vi "Launcher.vi"   [LabVIEW 2019]
uses:
  #typedef_LauncherStates_enum.ctl
  #typedef_Queue_enum.ctl
  #typedef_Data_Entry.ctl
  #typedef_EntryConsole_Action_enum.ctl
  #typedef_Data_Cluster.ctl
  #typedef_WashDisplay_Action_enum.ctl
  #typedef_Controller_Action_enum.ctl
  #typedef_VehiclePosition_Action_enum.ctl
  #typedef_Data_Controller.ctl
types:
  T1 = typedef "#typedef_LauncherStates_enum.ctl" = enum16{"ERROR_default", "DefineCustomError", "InitIntermoduleQueues", "InitModules", "Run", "CloseIntermoduleQueues", "CloseApp"}
  T2 = typedef "#typedef_Queue_enum.ctl" = enum16{"ERROR_default", "Obtain", "Enqueue", "GetStatus", "Flush", "Release"}
  T3 = typedef "#typedef_Data_Controller.ctl" = cluster{"EntryConsole_Action":T4, "WashDisplay_Action":T5, "Controller_Action":T6, "VehiclePosition_Action":T7}
  T4 = typedef "#typedef_EntryConsole_Action_enum.ctl" = enum16{"Init", "ERROR_DEFAULT", "Idle", "Pending_Wash_Cycle", "Clear_Console", "Close", "Error_Handler", "Exit"}
  T5 = typedef "#typedef_WashDisplay_Action_enum.ctl" = enum16{"Init", "ERROR_DEFAULT", "Idle", "Specific", "Close", "Error_Handler", "Exit"}
  T6 = typedef "#typedef_Controller_Action_enum.ctl" = enum16{"Init", "ERROR_DEFAULT", "Idle", "Read database", "Close", "Error_Handler", "Exit"}
  T7 = typedef "#typedef_VehiclePosition_Action_enum.ctl" = enum16{"Init", "ERROR_DEFAULT", "Idle", "Specific", "Close", "Error_Handler", "Exit"}
  T8 = typedef "#typedef_Data_Cluster.ctl" = cluster{"Dummy":dbl, "EntryConsole_Action":T4, "WashDisplay_Action":T5, "Controller_Action":T6, "VehiclePosition_Action":T7}
  T9 = typedef "#typedef_Data_Entry.ctl" = cluster{"Under Body Wash":bool, "Bug Remover":bool, "Pre-Soak":bool, "High Pressure Wash (default)":bool, "Low Pressure Wax":bool, "Spot Free Rinse":bool, "Tire Shine Foam":bool, "Air Dry":bool, "Start":bool, "EntryConsole_Action":T4}
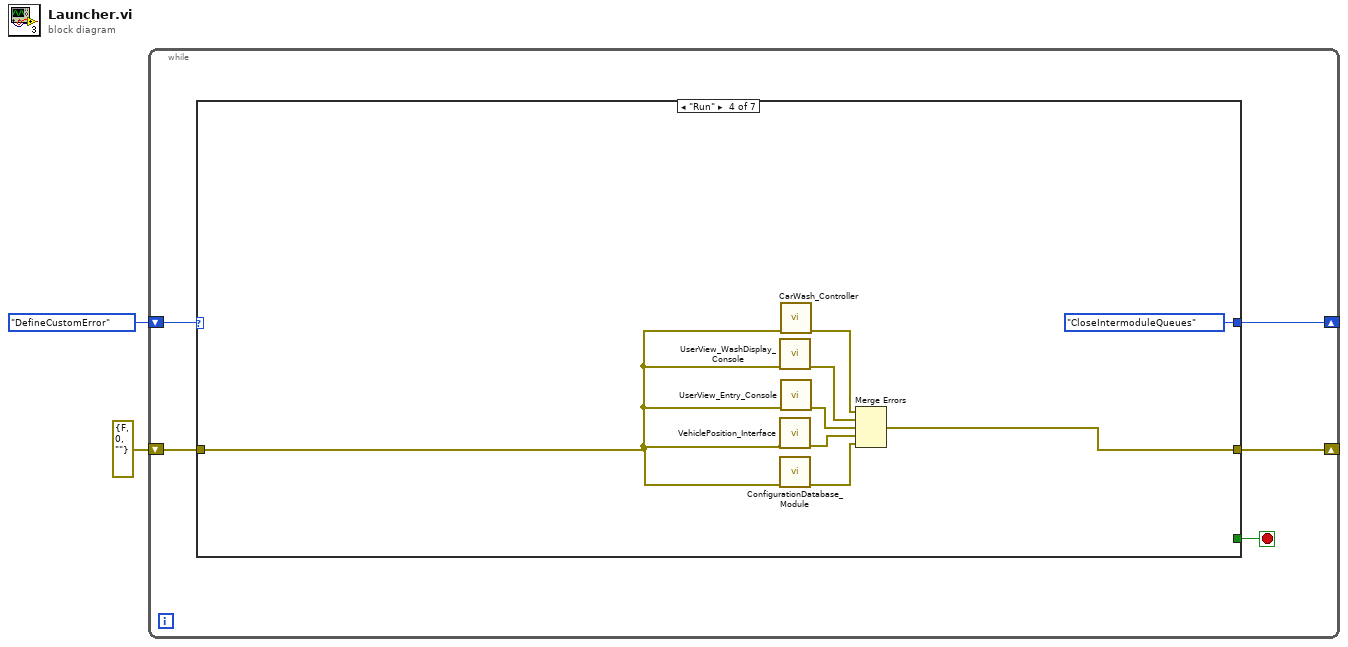
[diagram p0: block diagram]
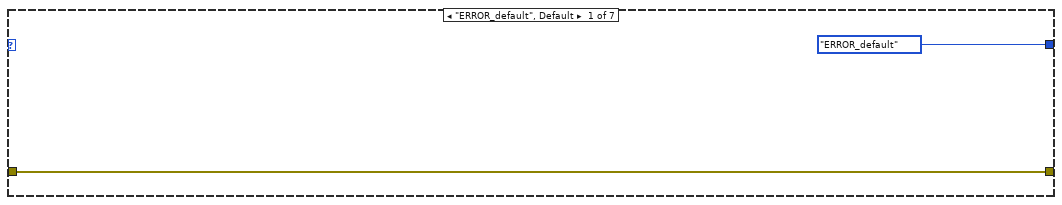
[diagram p2: hidden frame]
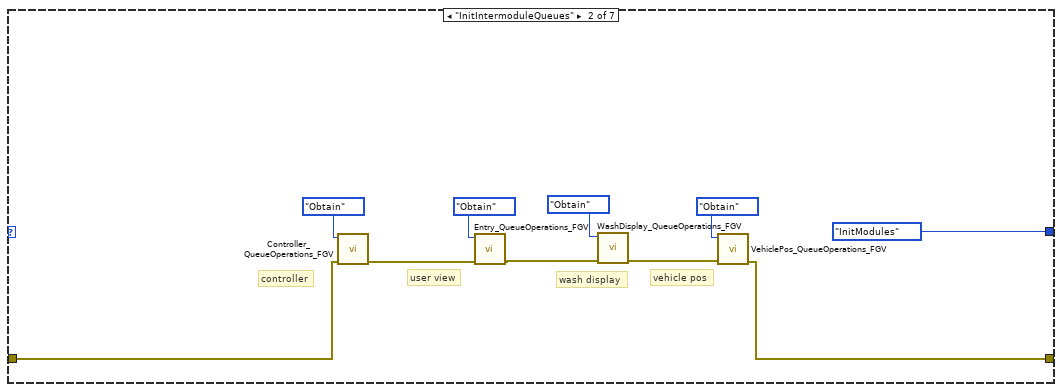
[diagram p3: hidden frame]
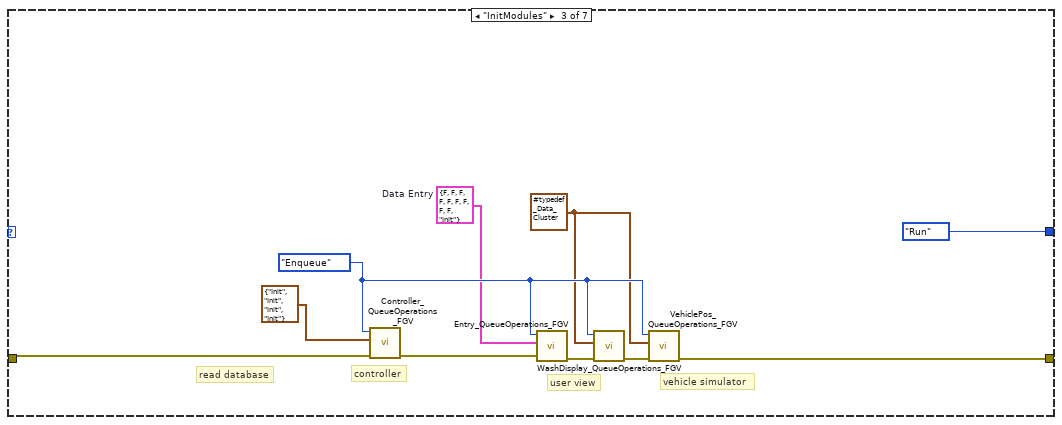
[diagram p4: hidden frame]
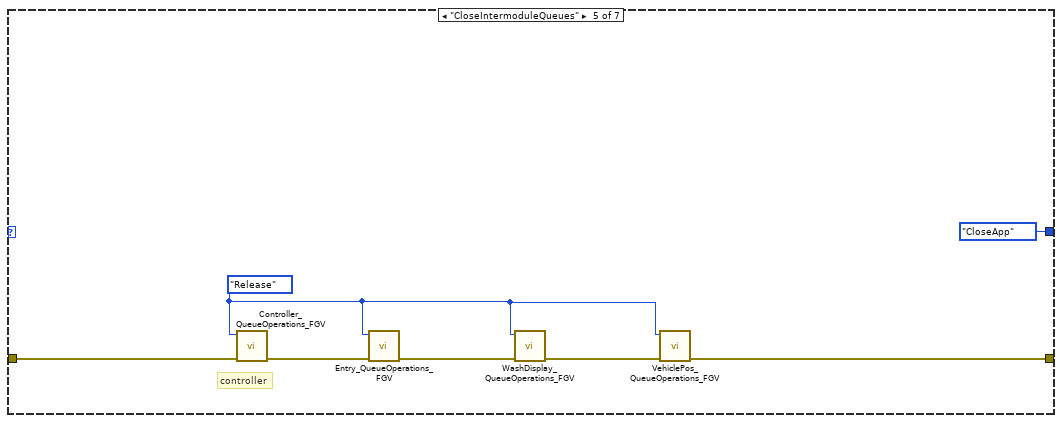
[diagram p5: hidden frame]
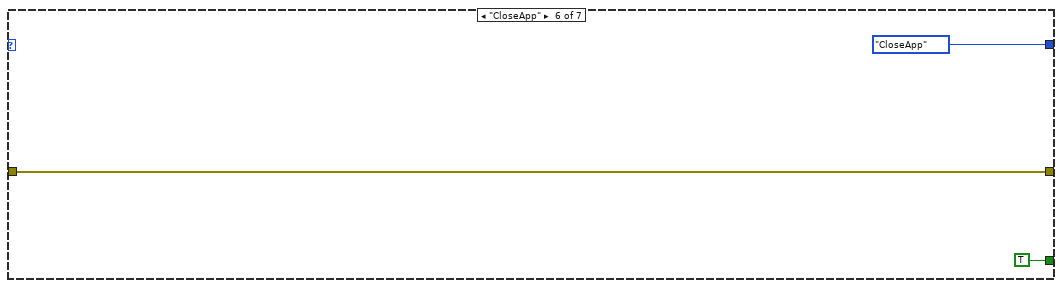
[diagram p6: hidden frame]
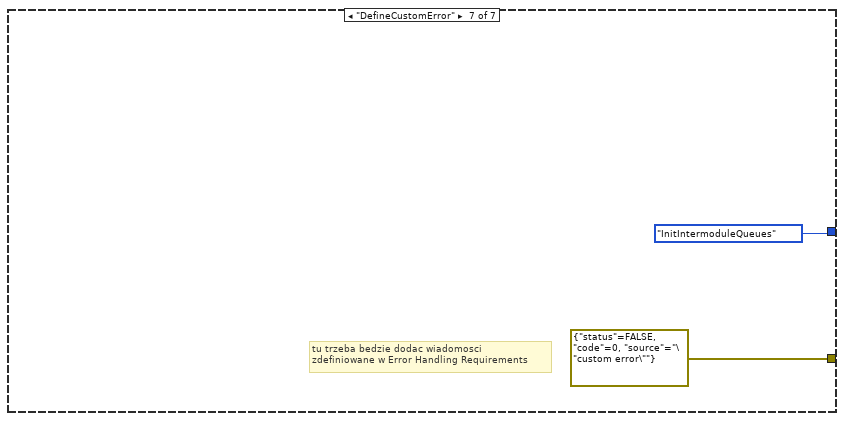
[diagram p7: hidden frame]
diagram:
  n1 = while {
    shift-right: [w5] -> _
    shift-left: #typedef_LauncherStates_enum."DefineCustomError" -> [w7]
    shift-right: [w6] -> _
    shift-left: errorcluster {"status"=FALSE, "code"=0, "source"=""} ("error constant") -> [w3]
    stop <- w4 stop-if-true
    n2 = case shown="\"Run\"" w7 {
      tunnel: w3 -> [w8 w18 w28 w32 w44 w45 _]
      tunnel: [w8 w15 w24 w31 w40 w45 errorcluster {"status"=FALSE, "code"=0, "source"="\"custom error\""} ("error constant")] -> w6
      tunnel: [#typedef_LauncherStates_enum."ERROR_default" #typedef_LauncherStates_enum."InitModules" #typedef_LauncherStates_enum."Run" #typedef_LauncherStates_enum."CloseIntermoduleQueues" #typedef_LauncherStates_enum."CloseApp" #typedef_LauncherStates_enum."CloseApp" #typedef_LauncherStates_enum."InitIntermoduleQueues"] -> w5
      tunnel: [_ _ _ _ _ TRUE _] -> w4
      frame "ERROR_default", Default {
      }
      frame "InitIntermoduleQueues" {
        # "wash display"
        # "vehicle pos"
        # "user view"
        # "controller"
        n3 = call "Controller_QueueOperations_FGV.vi"("error in"=w18, "Action"=#typedef_Queue_enum."Obtain") -> ("error out"=w19:errorcluster)  [unwired: 6 in, 3 out]
        n4 = call "Entry_QueueOperations_FGV.vi"("error in"=w19, "Action"=#typedef_Queue_enum."Obtain") -> ("error out"=w16:errorcluster)  [unwired: 6 in, 3 out]
        n5 = call "WashDisplay_QueueOperations_FGV.vi"("error in"=w16, "Action"=#typedef_Queue_enum."Obtain") -> ("error out"=w11:errorcluster)  [unwired: 6 in, 3 out]
        n6 = call "VehiclePos_QueueOperations_FGV.vi"("error in"=w11, "Action"=#typedef_Queue_enum."Obtain") -> ("error out"=w15:errorcluster)  [unwired: 6 in, 3 out]
      }
      frame "InitModules" {
        w21 = T8 {"Dummy"=0.0, "EntryConsole_Action"=enum."Init", "WashDisplay_Action"=enum."Init", "Controller_Action"=enum."Init", "VehiclePosition_Action"=enum."Init"} ("Data")
        w22 = T9 {"Under Body Wash"=FALSE, "Bug Remover"=FALSE, "Pre-Soak"=FALSE, "High Pressure Wash (default)"=FALSE, "Low Pressure Wax"=FALSE, "Spot Free Rinse"=FALSE, "Tire Shine Foam"=FALSE, "Air Dry"=FALSE, "Start"=FALSE, "EntryConsole_Action"=enum."Init"}  # Data Entry
        w23 = #typedef_Queue_enum."Enqueue" ("Action")
        # "vehicle simulator"
        # "user view"
        # "controller"
        # "read database"
        n7 = call "Controller_QueueOperations_FGV.vi"("error in"=w28, "Data In"=T3 {"EntryConsole_Action"=enum."Init", "WashDisplay_Action"=enum."Init", "Controller_Action"=enum."Init", "VehiclePosition_Action"=enum."Init"} ("Data"), "Action"=w23) -> ("error out"=w26:errorcluster)  [unwired: 5 in, 3 out]
        n8 = call "Entry_QueueOperations_FGV.vi"("error in"=w26, "Data"=w22, "Action"=w23) -> ("error out"=w27:errorcluster)  [unwired: 5 in, 3 out]
        n9 = call "WashDisplay_QueueOperations_FGV.vi"("error in"=w27, "Data"=w21, "Action"=w23) -> ("error out"=w25:errorcluster)  [unwired: 5 in, 3 out]
        n10 = call "VehiclePos_QueueOperations_FGV.vi"("error in"=w25, "Data"=w21, "Action"=w23) -> ("error out"=w24:errorcluster)  [unwired: 5 in, 3 out]
      }
      frame "Run" {
        n11 = call "UserView_WashDisplay_Console.vi"("error in"=w32) -> ("error out"=w33:errorcluster)  [unwired: 10 in]
        n12 = call "VehiclePosition_Interface.vi"("error in"=w32) -> ("error out"=w36:errorcluster)  [unwired: 10 in]
        n13 = call "ConfigurationDatabase_Module.vi"("error in"=w32) -> ("error out"=w35:errorcluster)  [unwired: 9 in, 1 out]
        n14 = call "CarWash_Controller.vi"("error in"=w32) -> ("error out"=w34:errorcluster)  [unwired: 10 in]
        n15 = call "UserView_Entry_Console.vi"("error in"=w32) -> ("error out"=w37:errorcluster)  [unwired: 10 in]
        n16 = Merge Errors(w34, w33, w37, w36, w35) -> (w31:errorcluster)
      }
      frame "CloseIntermoduleQueues" {
        w39 = #typedef_Queue_enum."Release" ("Action")
        # "controller"
        n17 = call "Controller_QueueOperations_FGV.vi"("error in"=w44, "Action"=w39) -> ("error out"=w43:errorcluster)  [unwired: 6 in, 3 out]
        n18 = call "Entry_QueueOperations_FGV.vi"("error in"=w43, "Action"=w39) -> ("error out"=w42:errorcluster)  [unwired: 6 in, 3 out]
        n19 = call "WashDisplay_QueueOperations_FGV.vi"("error in"=w42, "Action"=w39) -> ("error out"=w41:errorcluster)  [unwired: 6 in, 3 out]
        n20 = call "VehiclePos_QueueOperations_FGV.vi"("error in"=w41, "Action"=w39) -> ("error out"=w40:errorcluster)  [unwired: 6 in, 3 out]
      }
      frame "CloseApp" {
      }
      frame "DefineCustomError" {
        # "tu trzeba bedzie dodac wiadomosci\nzdefiniowane w Error Handling Requirements"
      }
    }
  }
